vi "picoquant_write_data_logger.vi"(8 "error in (no error)":errorcluster, 10 "data_logger.lvclass":refnum<class "data_logger.lvclass">, 11 "picoharp in":refnum<class "picoharp.lvclass">) -> (0 "error out":errorcluster, 3 "picoharp out":refnum<class "picoharp.lvclass">)   [LabVIEW 2015, in "picoharp.lvclass"]
uses:
  picoharp.lvclass
  Data Logger Class/data_logger.lvclass
  picoharp.lvclass/picoharp.ctl
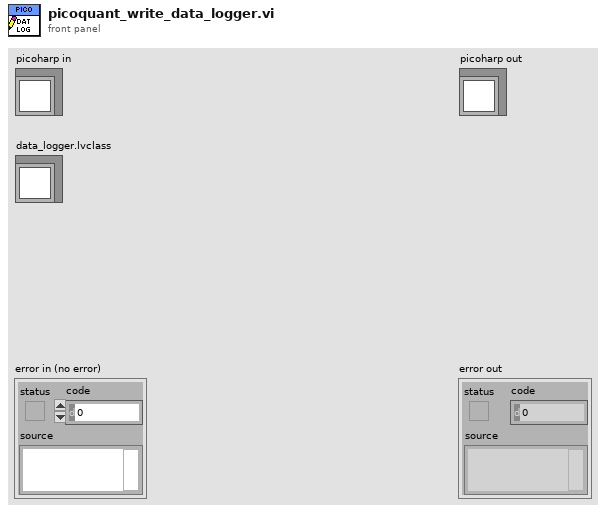
[diagram p1: front panel]
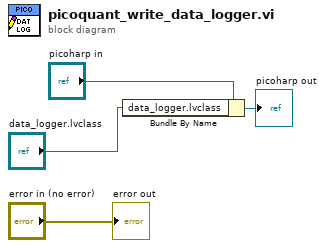
[diagram p0: block diagram]
diagram:
  n1 = Bundle By Name(cluster="picoharp in", "data_logger.lvclass"="data_logger.lvclass") -> (→"picoharp out":refnum<class "picoharp.lvclass">)
  "error out" <- "error in (no error)"
